vi "Grab_Function.vi"(9 "cameraId":u32) -> (1 "output cluster":T1, 3 "imgPtr":i32[][](array[numeric]))   [LabVIEW 2017, in "PlayNitrideCameraComponet1010_4.lvlib"]
uses:
  <userlib>/PlayNitrideCameraComponet1010_4/PlayNitrideCameraComponet1010_4.lvlib
panel:
  in  "ImageSize":T1
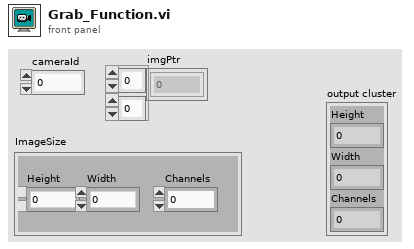
[diagram p1: front panel]
types:
  T1 = cluster{"Height":dbl, "Width":dbl, "Channels":dbl}
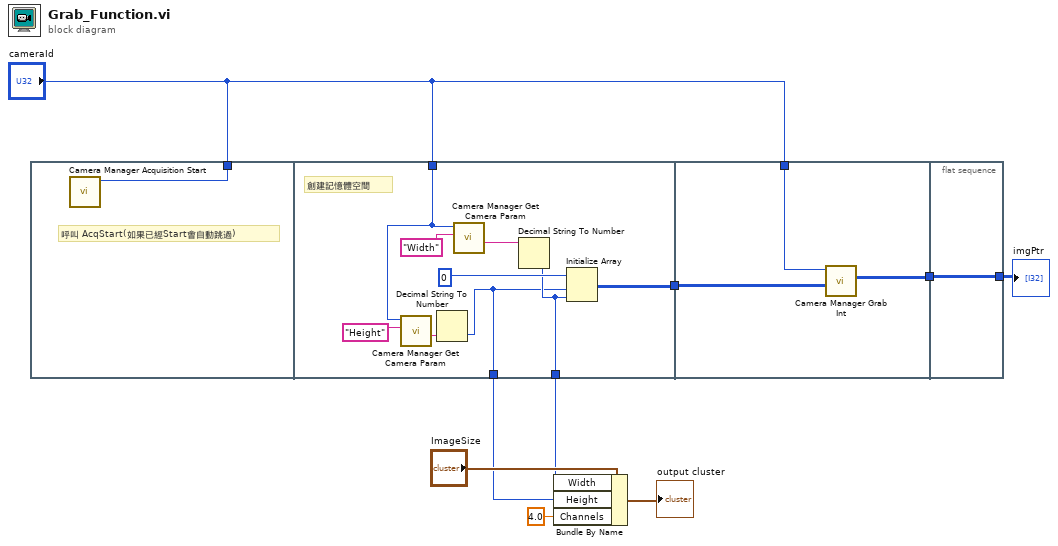
[diagram p0: block diagram]
diagram:
  n1 = flat-sequence {
    tunnel: "cameraId" -> [w10]
    tunnel: [w18] -> w9
    tunnel: "cameraId" -> [w11]
    tunnel: [w17] -> w4
    tunnel: [w16] -> w3
    tunnel: "cameraId" -> [w22]
    tunnel: w9 -> [w20]
    tunnel: [w21] -> w7
    tunnel: [w23] -> w6
    tunnel: w7 -> [w23]
    frame #0 {
      # "呼叫 AcqStart(如果已經Start會自動跳過)"
      n2 = call <userlib>:"Camera Manager Acquisition Start.vi"("cameraId"=w10) -> ()  [unwired: 10 in, 1 out]
    }
    frame #1 {
      # "創建記憶體空間"
      n3 = call <userlib>:"Camera Manager Get Camera Param.vi"("NodeName"="Height", "cameraId"=w11) -> ("Value out"=w13:string)  [unwired: 7 in, 2 out]
      n4 = Decimal String To Number(string=w13) -> (number=w16:i32)  [unwired: 2 in, 1 out]
      n5 = call <userlib>:"Camera Manager Get Camera Param.vi"("NodeName"="Width", "cameraId"=w11) -> ("Value out"=w15:string)  [unwired: 7 in, 2 out]
      n6 = Decimal String To Number(string=w15) -> (number=w17:i32)  [unwired: 2 in, 1 out]
      n7 = Initialize Array(u32 0 ("unsigned 32bit integer"), w16, w17) -> (w18:u32[][])
    }
    frame #2 {
      n8 = call <userlib>:"Camera Manager Grab Int.vi"("imgPtr Input"=w20, "cameraId"=w22) -> ("imgPtr"=w21:i32[][])  [unwired: 8 in, 1 out]
    }
    frame #3 {
    }
  }
  n9 = Bundle By Name(cluster="ImageSize", "Width"=w4, "Height"=w3, "Channels"=4.0) -> (→"output cluster":T1)
  "imgPtr" <- w6
